vi "Top level VI V2.vi"() -> ()   [LabVIEW 2014]
uses:
  <vilib>/Platform/TimedLoop/XDataNode/timing_clust.ctl
  <vilib>/Platform/TimedLoop/XDataNode/nitl_modes.ctl
  <vilib>/Platform/TimedLoop/XDataNode/wakeup.ctl
  <vilib>/rvi/Emulation/niFpgaGetClockAttributes.vi
  <vilib>/rvi/Emulation/niFpgaSctlEmulationGetInTimedLoop.vi
  <vilib>/rvi/Emulation/niFpgaEmulationReportErrorSimple.vi
  <vilib>/rvi/eio/common/nirviEmuTemplateMethod_errors.vi
  <vilib>/rvi/Emulation/niFpgaEmulationIsFPGAContextNoSignature.vi
  <vilib>/rvi/errors/niFpgaSetErrorForExecOnDevCompSimple.vi
  <vilib>/rvi/eio/common/nirviEmuReportErrorAndStop.vi
  <vilib>/rvi/DataTransferAndStorage/Container/Common/niFpgaContainerGetUniqueNameForEmu.vi
  <vilib>/rvi/FIFO/Fifo_Resource/nirvififoEmulationSetSize.vi
  <vilib>/rvi/FIFO/Fifo_Resource/nirviFifoEmulationQueueMgr.vi
  <instcachedir>/0/nirviFifoEmulationQueueMgr_E5CAEC123FF24DC58D834DCA3CDAA9B5.lvgen/nirviFifoEmulationQueueMgr_E5CAEC123FF24DC58D834DCA3CDAA9B5_002.vi
  <vilib>/rvi/FIFO/Fifo_Resource/nirvififoEmulationDetermineInputValidOut.vi
  <vilib>/rvi/FIFO/Fifo_Resource/nirvififoEmulationCreateLock.vi
  <vilib>/rvi/Emulation/niFpgaProcessEmulError.vi
  <vilib>/rvi/FIFO/Fifo_Resource/nirvififoEmulationObtainLock.vi
  <vilib>/rvi/FIFO/Fifo_Resource/nirvififoEmulationReleaseLock.vi
  <vilib>/rvi/occurrence/nirviWaitOnOccurrenceBase.vi
  <vilib>/rvi/errors/nirviReportUnexpectedCaseInternalError.vi
  <vilib>/rvi/errors/nirviReportUnexpectedCaseInternalError (U32).vi
  <vilib>/rvi/Memory/Memory_Emulation/nirvimemoryEmulation.vi
  <vilib>/rvi/Memory/Memory_Emulation/nirvimemoryFastEmulation.vi
  <vilib>/rvi/Memory/Memory_Emulation/niFpgaMemoryEmulationCacheClearOnFirstRun.vi
  <vilib>/rvi/Memory/Memory_Emulation/nirvimemoryEmulationManagerCache_MakeExclusive.vi
  <vilib>/rvi/Memory/Memory_Emulation/niFpgaMemoryEmulationValidateCache.vi
  <vilib>/rvi/Memory/Memory_Emulation/nirvimemoryEmulationManagerCache_InsertValue.vi
  <vilib>/Utility/error.llb/Clear Errors.vi
  <vilib>/rvi/Memory/Memory_Emulation/nirvimemoryEmulationManagerCache_ReleaseExclusive.vi
  <vilib>/rvi/Memory/Memory_Emulation/nirvimemoryEmulationManagerCache_GetValue.vi
  <vilib>/rvi/Memory/Memory_Emulation/nirvimemoryEmulationManagerCache_SetValue.vi
  <vilib>/rvi/Emulation/niFpgaSctlEmulationResourceMgr.vi
  <vilib>/rvi/Emulation/niFpgaCriticalErrorInLSC.vi
  <vilib>/rvi/interface/RandomDataEmulation/niFpgaRandomDataHandleErrors.vi
  <vilib>/eio/EIOMethodNode/EIOMethodNode.xnode
  <vilib>/rvi/DataTransferAndStorage/Container/XNode/niFpgaContainer.xnode
  <vilib>/rvi/FIFO/Fifo_Resource/nirvififoEmulationWrite.vi
  <vilib>/Platform/TimedLoop/XDataNode/XDataNode.xnode
  <vilib>/rvi/FIFO/Fifo_Resource/nirvififoEmulationGetNumberOfElementsToRead.vi
  <vilib>/rvi/FIFO/Fifo_Resource/nirvififoEmulationRead.vi
  <vilib>/rvi/interface/RandomDataEmulation/nirviRandomDataFpgaReadWriteTemplate.vi
  <vilib>/Platform/TimedLoop/XDataNode/XDNodeRunTimeDep.lvlib
panel:
  out "Execution Time":u32
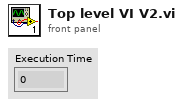
[diagram p1: front panel]
types:
  T1 = typedef "XDNodeRunTimeDep.lvlib/timing_clust.ctl" = cluster{"Expected End [f-1]":u64, "Actual End [f-1]":u64, "Finished Late? [f-1]":bool, "Expected End [i-1]":u64, "Actual End [i-1]":u64, "Finished Late? [i-1]":bool, "Expected Start [i]":u64, "Actual Start [i]":u64, "Expected Start [f]":u64, "Actual Start [f]":u64, "Source Name":string, "Structure Name":string, "Period":i64, "Deadline":i64, "Offset":i64, "Start":i64, "Priority":i32, "Timeout":i32, "Mode":T2, "Wakeup Reason":T3, "Error":errorcluster, "Source Type":string, "Secondary Source Type":string, "Global End Time":u64, "Global Start Time":u64, "Frame Duration":u64, "Iteration Duration":u64, "Assigned CPU":i32, "I/O Scan Engine Mode":u32}
  T2 = typedef "XDNodeRunTimeDep.lvlib/nitl_modes.ctl" = enum32{"No Change", "Process missed periods, maintain original phase", "Discard missed periods, maintain original phase", "Process missed periods, ignore original phase", "Discard missed periods, ignore original phase"}
  T3 = typedef "XDNodeRunTimeDep.lvlib/wakeup.ctl" = enum32{"Normal", "Aborted", "Asynchronous wakeup", "Timing source error", "Timed loop error", "Timeout"}
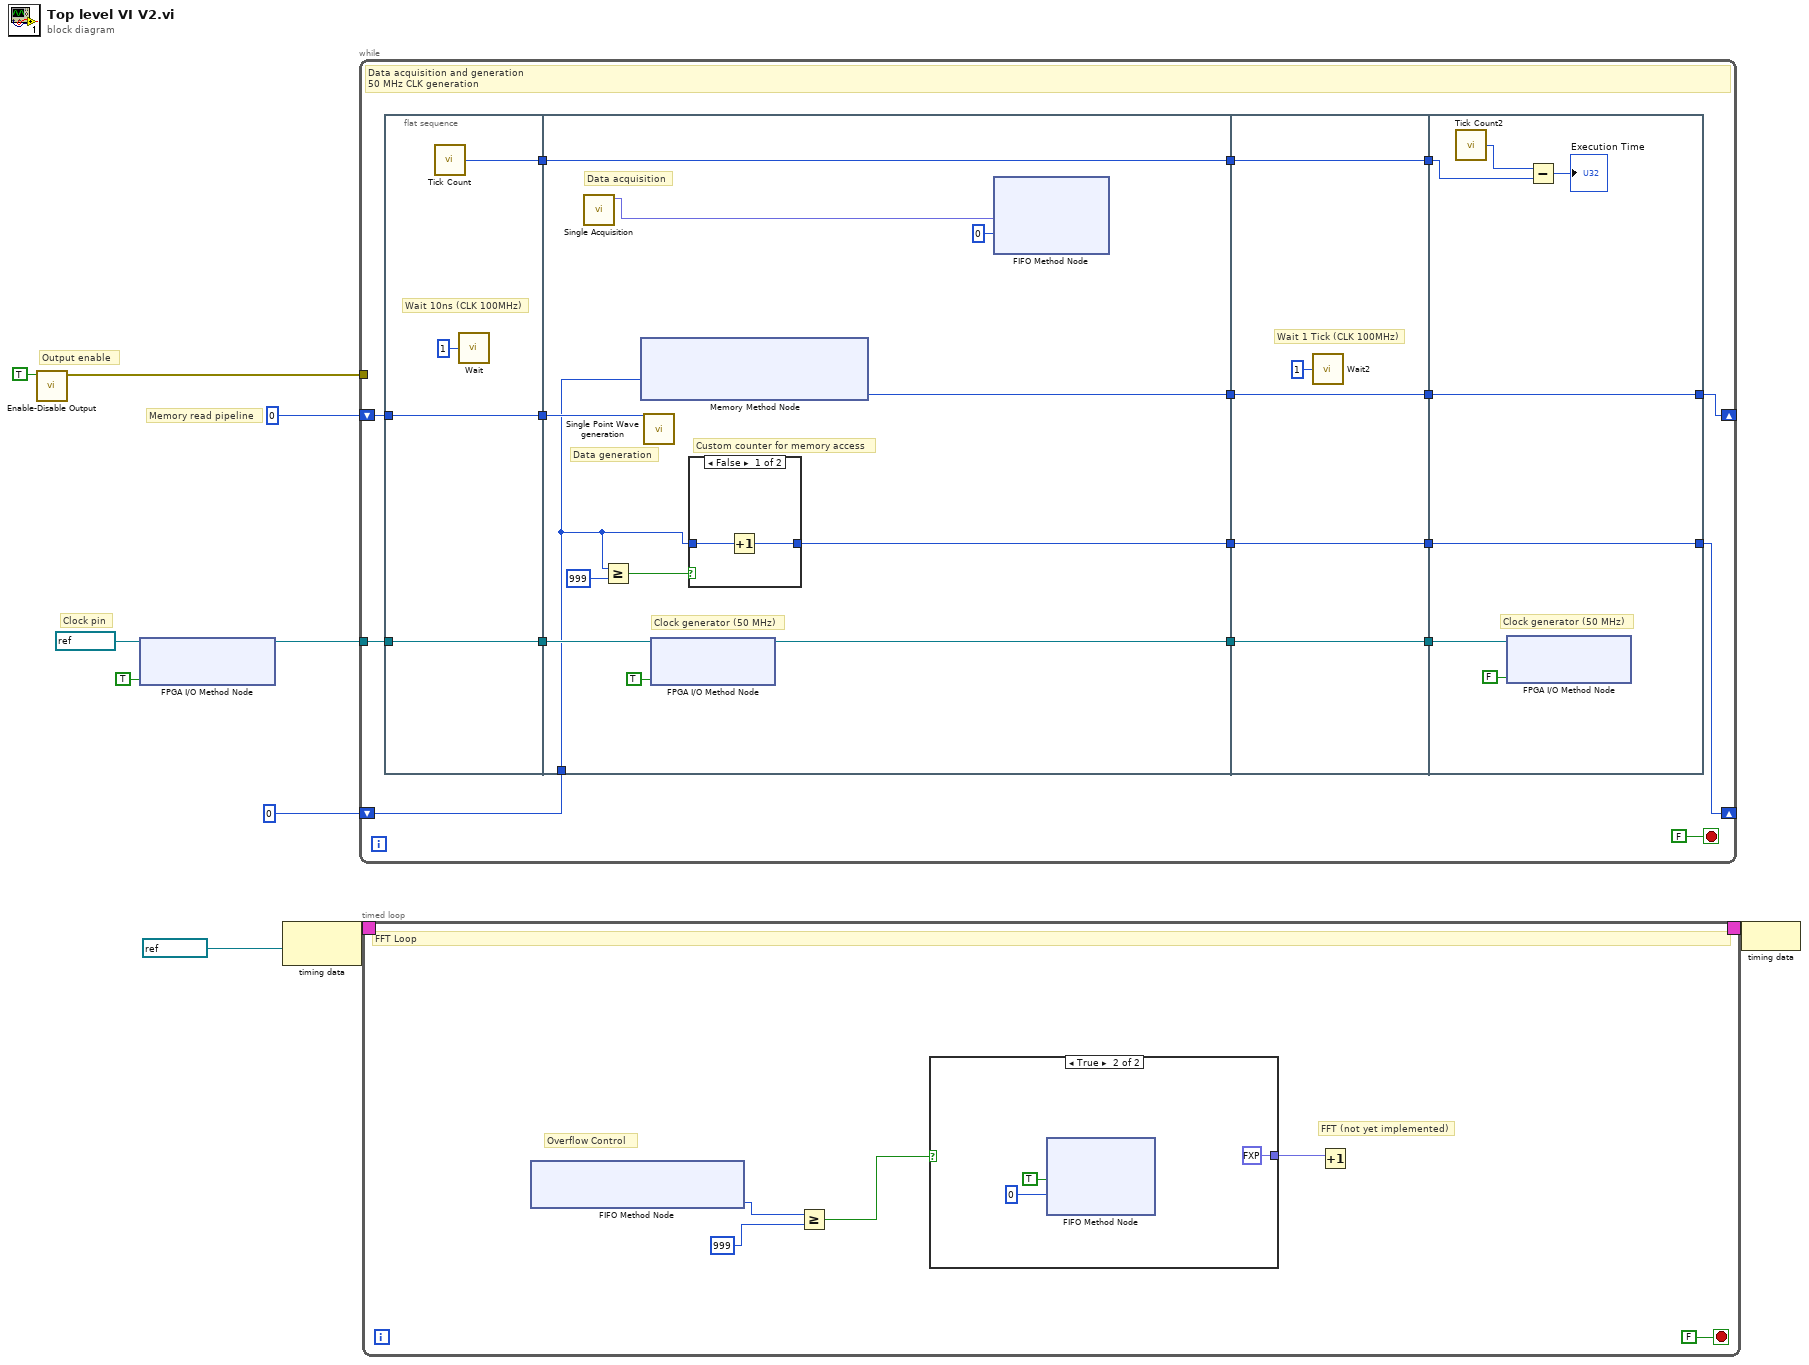
[diagram p0: block diagram]
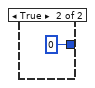
[diagram p2: hidden frame]
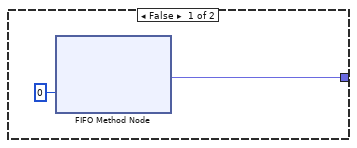
[diagram p3: hidden frame]
diagram:
  # "Memory read pipeline"
  # "Clock pin"
  # "Output enable"
  n1 = call "Enable-Disable Output.vi"("Enable"=TRUE) -> ("error out"=w4:errorcluster)  [unwired: 10 in]
  n2 = xnode "FPGA I/O Method Node"("FPGA I/O In"=refnum<k21> "DIO24", "Enable"=TRUE) -> ("FPGA I/O Out"=w8:refnum<k21>)
  n3 = node-c288(refnum<k21> "50MHz" ("Source Name")) -> (w3:T1)
  n4 = while {
    tunnel: w8 -> [w24]
    shift-right: [w17] -> _
    shift-left: i16 0 -> [w20]
    shift-right: [w15] -> _
    shift-left: u32 0 -> [w16]
    tunnel: w4 -> [_]
    stop <- FALSE stop-if-true
    # "Data acquisition and generation\n50 MHz CLK generation"
    n5 = flat-sequence {
      tunnel: [w30] -> w25
      tunnel: w24 -> [w30]
      tunnel: [w29] -> w21
      tunnel: w20 -> [w29]
      tunnel: [w28] -> w11
      tunnel: [w41] -> w27
      tunnel: w25 -> [w39]
      tunnel: [w37] -> w22
      tunnel: w21 -> [w36]
      tunnel: [w35] -> w18
      tunnel: w16 -> [w34]
      tunnel: [w32] -> w12
      tunnel: w11 -> [w32]
      tunnel: w27 -> [w51]
      tunnel: [w51] -> w26
      tunnel: [w49] -> w23
      tunnel: w22 -> [w49]
      tunnel: [w48] -> w19
      tunnel: w18 -> [w48]
      tunnel: [w47] -> w13
      tunnel: w12 -> [w47]
      tunnel: [w58] -> w15
      tunnel: w26 -> [w58]
      tunnel: w23 -> [w57]
      tunnel: [w55] -> w17
      tunnel: w19 -> [w55]
      tunnel: w13 -> [w53]
      frame #0 {
        # "Wait 10ns (CLK 100MHz)"
        n6 = call "Tick Count"() -> ("Tick Count(mSec)"=w28:u32)
        n7 = call "Wait"("Count(Ticks)"=u8 1) -> ()  [unwired: 1 out]
      }
      frame #1 {
        # "Data generation"
        # "Custom counter for memory access"
        # "Clock generator (50 MHz)"
        # "Data acquisition"
        n8 = call "Single Acquisition.vi"() -> ("fixed-point"=w40:fxp<+/-,12,5>)  [unwired: 11 in]
        n9 = Greater Or Equal?(x=w34, y=u32 999) -> (x >= y?=w42:bool)
        n10 = xnode ("Memory Method Node")("Address"=w34) -> ("Data"=w35:i16)  [unwired: 1 in, 1 out]
        n11 = call "Single Point Wave generation.vi"("Data To Write"=w36) -> ()  [unwired: 10 in, 1 out]
        n12 = xnode "FPGA I/O Method Node"("FPGA I/O In"=w39, "Data"=TRUE) -> ("FPGA I/O Out"=w37:refnum<k21>)
        n13 = case shown="False" w42 {
          tunnel: w34 -> [w45 _]
          tunnel: [w44 0] -> w41
          frame False {
            n14 = Increment(x=w45) -> (x+1=w44:u32)
          }
          frame True {
          }
        }
        n15 = xnode ("FIFO Method Node")("Element"=w40, "Timeout"=0) -> ()  [unwired: 1 in, 2 out]
      }
      frame #2 {
        # "Wait 1 Tick (CLK 100MHz)"
        n16 = call "Wait2"("Count(Ticks)"=u8 1) -> ()  [unwired: 1 out]
      }
      frame #3 {
        # "Clock generator (50 MHz)"
        n17 = call "Tick Count2"() -> ("Tick Count(mSec)"=w54:u32)
        n18 = xnode "FPGA I/O Method Node"("FPGA I/O In"=w57, "Data"=FALSE) -> ()  [unwired: 1 out]
        n19 = Subtract(x=w54, y=w53) -> (x-y=→"Execution Time":u32)
      }
    }
  }
  n20 = timed-loop {
    timing: w3 -> [_]
    timing-out: [_] -> w2
    stop <- FALSE stop-if-true
    # "FFT (not yet implemented)"
    # "Overflow Control"
    # "FFT Loop"
    n21 = xnode ("FIFO Method Node")() -> ("Number of Elements to Read"=w63:u32)  [unwired: 1 in, 1 out]
    n22 = Greater Or Equal?(x=w63, y=u32 999) -> (x >= y?=w61:bool)
    n23 = case shown="True" w61 {
      tunnel: [w64 fxp<+/-,12,5> 0.0 ("Element")] -> w60
      frame False {
        n24 = xnode ("FIFO Method Node")("Timeout"=0) -> ("Element"=w64:fxp<+/-,12,5>)  [unwired: 1 in, 2 out]
      }
      frame True {
        n25 = xnode ("FIFO Method Node")("Element"=TRUE, "Timeout"=0) -> ()  [unwired: 1 in, 2 out]
      }
    }
    n26 = Increment(x=w60) -> ()  [unwired: 1 out]
  }
  n27 = node-c288(w2) -> ()
